vi "motor_cleanup.vi"(4 "error in (no error)":errorcluster, 6 "Request data":variant, 7 "Python session in":refnum<k35>) -> (0 "error out":errorcluster, 2 "Response data":variant, 3 "Python session out":refnum<k35>)   [LabVIEW 2022 SP3]
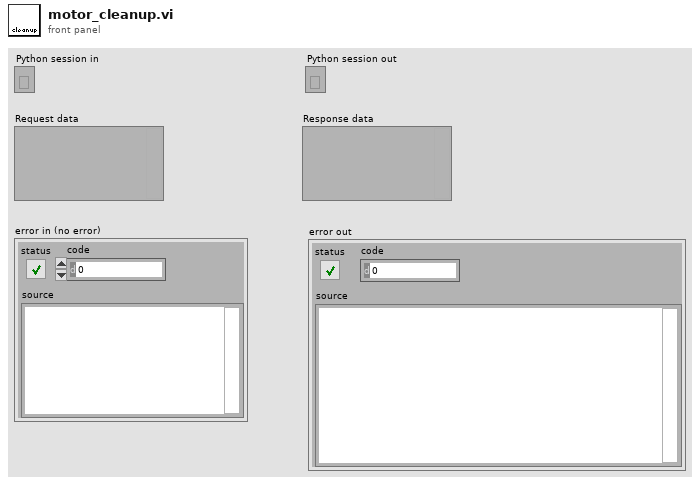
[diagram p1: front panel]
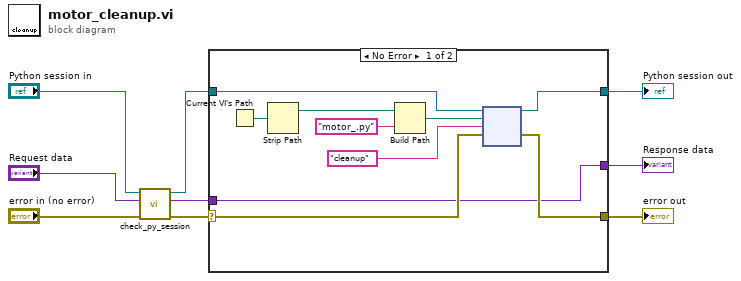
[diagram p0: block diagram]
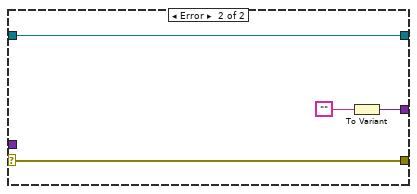
[diagram p2: hidden frame]
diagram:
  n1 = call "check_py_session.vi"("error in"="error in (no error)", "Request data"="Request data", "Python session in"="Python session in") -> ("error out"=w3:errorcluster, "Response data"=w4:variant, "Python session out"=w5:refnum<k35>)  [unwired: 2 in]
  n2 = case shown="No Error" w3 {
    selector: w3 -> [w11 w23]
    tunnel: w5 -> [w19 w22]
    tunnel: [w13 w22] -> w9
    tunnel: w4 -> [w10 _]
    tunnel: [w12 w23] -> w2
    tunnel: [w10 w20] -> w1
    frame No Error {
      n3 = Current VI's Path() -> (path=w15:path)
      n4 = Strip Path(path=w15) -> (stripped path=w14:path)  [unwired: 1 out]
      n5 = Build Path(base path=w14, name or relative path="motor_.py") -> (appended path=w17:path)
      n6 = node(w19, w17, "cleanup" ("function name"), w11) -> (w13:refnum<k35>, w12:errorcluster)  [unwired: 2 in, 2 out]
    }
    frame Error {
      n7 = To Variant(anything="") -> (Variant=w20:variant)
    }
  }
  "error out" <- w2
  "Python session out" <- w9
  "Response data" <- w1
